vi "identity.vi"(8 "error in":errorcluster, 11 "Identity":T1 {"type" items=["Client", "Service"]}) -> (0 "error out":errorcluster, 3 "JSON Tree out (JSON Object)":variant)   [LabVIEW 2010]
uses:
  i3-json-1.0.0-10/JSON Generation/Create Value Files/Create Value - Object.vi
  i3-json-1.0.0-10/JSON Generation/Add Object Parameter Files/Add Object Parameter - String.vi
  i3-json-1.0.0-10/JSON Generation/Add Object Parameter Files/Add Object Parameter - Object.vi
  i3-json-1.0.0-10/i3-json.lvlib
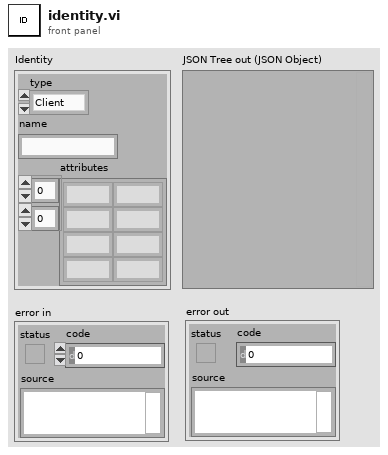
[diagram p1: front panel]
types:
  T1 = cluster{"type":u16, "name":string, "attributes":string[][]}
  T2 = enum32{"invalid CPU target", "Motorola 68K", "PowerPC", "Intel x86", "SPARC", "PA-RISC", "MIPS", "Alpha", "ARM", "AMD/Intel x64"}
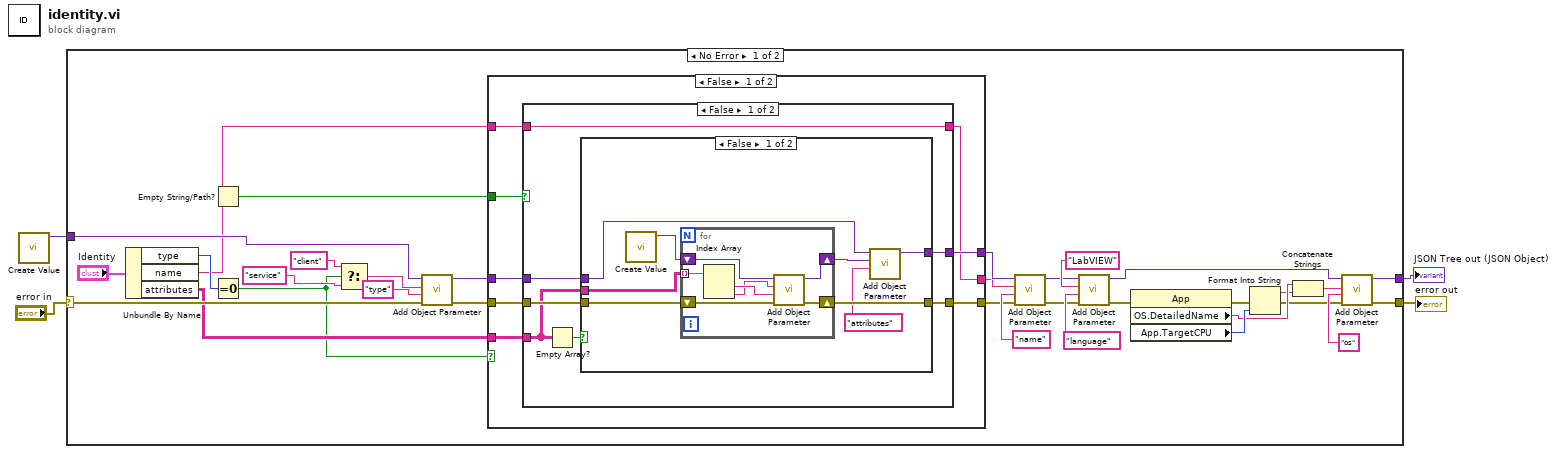
[diagram p0: block diagram]
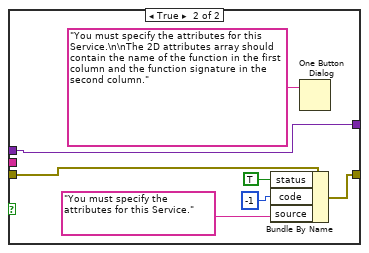
[diagram p2: hidden frame]
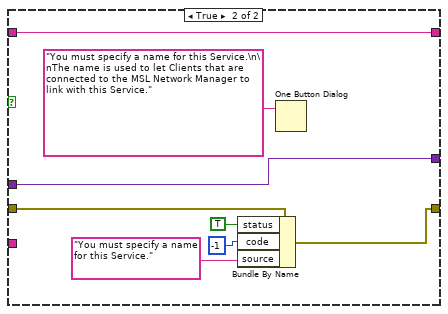
[diagram p3: hidden frame]
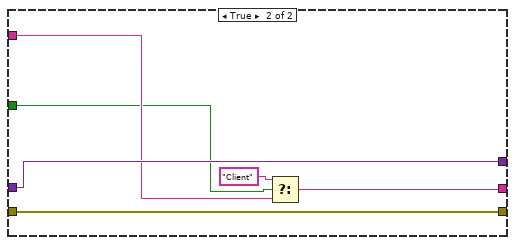
[diagram p4: hidden frame]
diagram:
  n1 = call-poly "Create Value.vi"() -> ("JSON Tree"=w3:variant)  [unwired: 10 in, 1 out]
  n2 = case shown="No Error" "error in" {
    selector: "error in" -> [w28 w90]
    tunnel: [w29 w89] -> w4
    tunnel: [w11 w90] -> w1
    tunnel: w3 -> [w27 w89]
    frame No Error {
      n3 = Unbundle By Name("Identity") -> ("type"=w26:u16, "name"=w8:string, "attributes"=w20:string[][])
      n4 = Empty String/Path?(string/path=w8) -> (empty?=w6:bool)
      n5 = Equal To 0?(x=w26) -> (x = 0?=w9:bool)
      n6 = Select(t="client" ("language"), s=w9, f="service") -> (s? t:f=w22:string)
      n7 = call-poly "Add Object Parameter.vi"("error in (no error)"=w28, "Name"="type", "String"=w22, "JSON Tree in (JSON Object)"=w27) -> ("error out"=w21:errorcluster, "JSON Tree out (JSON Object)"=w19:variant)  [unwired: 6 in]
      n8 = case shown="False" w9 {
        tunnel: [w42 w88] -> w17
        tunnel: w21 -> [w45 w88]
        tunnel: w20 -> [w43 _]
        tunnel: w19 -> [w44 w87]
        tunnel: [w41 w87] -> w18
        tunnel: w8 -> [w38 w85]
        tunnel: [w39 w84] -> w7
        tunnel: w6 -> [w40 w83]
        frame False {
          n9 = case shown="False" w40 {
            tunnel: w45 -> [w52 w79]
            tunnel: w44 -> [w51 w78]
            tunnel: w43 -> [w50 _]
            tunnel: [w48 w77] -> w42
            tunnel: [w47 w78] -> w41
            tunnel: [w46 w76] -> w39
            tunnel: w38 -> [w46 w76]
            frame False {
              n10 = Empty Array?(array=w50) -> (empty?=w49:bool)
              n11 = case shown="False" w49 {
                tunnel: w52 -> [w60 w73]
                tunnel: w51 -> [w56 w69]
                tunnel: w50 -> [w59 _]
                tunnel: [w58 w70] -> w48
                tunnel: [w53 w69] -> w47
                frame False {
                  n12 = call-poly "Create Value.vi"() -> ("JSON Tree"=w57:variant)  [unwired: 10 in, 1 out]
                  n13 = for {
                    tunnel: w59 -> [w63] mode=indexing
                    shift-right: [w66] -> w54
                    shift-left: w57 -> [w67]
                    shift-right: [w64] -> w58
                    shift-left: w60 -> [w65]
                    n14 = Index Array(array=w63) -> (element #1=w62:string, element #2=w61:string)  [unwired: 2 in]
                    n15 = call-poly "Add Object Parameter.vi"("error in (no error)"=w65, "Name"=w62, "String"=w61, "JSON Tree in (JSON Object)"=w67) -> ("error out"=w64:errorcluster, "JSON Tree out (JSON Object)"=w66:variant)  [unwired: 6 in]
                  }
                  n16 = call-poly "Add Object Parameter.vi"("Name"="attributes" ("String"), "JSON Object"=w54, "JSON Tree in (JSON Object)"=w56) -> ("JSON Tree out (JSON Object)"=w53:variant)  [unwired: 7 in, 1 out]
                }
                frame True {
                  n17 = Bundle By Name(cluster=w73, "status"=TRUE, "code"=-1, "source"="You must specify the attributes for this Service." ("message")) -> (w70:errorcluster)
                  n18 = One Button Dialog(message="You must specify the attributes for this Service.\n\nThe 2D attributes array should contain the name of the function in the first column and the function signature in the second column.") -> ()  [unwired: 1 in, 1 out]
                }
              }
            }
            frame True {
              n19 = Bundle By Name(cluster=w79, "status"=TRUE, "code"=-1, "source"="You must specify a name for this Service." ("message")) -> (w77:errorcluster)
              n20 = One Button Dialog(message="You must specify a name for this Service.\n\nThe name is used to let Clients that are connected to the MSL Network Manager to link with this Service.") -> ()  [unwired: 1 in, 1 out]
            }
          }
        }
        frame True {
          n21 = Select(t="Client" ("language"), s=w83, f=w85) -> (s? t:f=w84:string)
        }
      }
      n22 = call-poly "Add Object Parameter.vi"("error in (no error)"=w17, "Name"="name", "String"=w7, "JSON Tree in (JSON Object)"=w18) -> ("error out"=w13:errorcluster, "JSON Tree out (JSON Object)"=w15:variant)  [unwired: 6 in]
      n23 = call-poly "Add Object Parameter.vi"("error in (no error)"=w13, "Name"="language", "String"="LabVIEW" ("language"), "JSON Tree in (JSON Object)"=w15) -> ("error out"=w12:errorcluster, "JSON Tree out (JSON Object)"=w33:variant)  [unwired: 6 in]
      n24 = property class="App"(error in=w12) -> (error out=w14:errorcluster, "OS.DetailedName"=w30:string, "App.TargetCPU"=w32:T2)  [unwired: 1 in, 1 out]
      n25 = Format Into String(error in=w14, w32) -> (resulting string=w5:string, error out=w10:errorcluster)  [unwired: 2 in]
      n26 = Concatenate Strings(w30, w5) -> (w31:string)
      n27 = call-poly "Add Object Parameter.vi"("error in (no error)"=w10, "Name"="os", "String"=w31, "JSON Tree in (JSON Object)"=w33) -> ("error out"=w11:errorcluster, "JSON Tree out (JSON Object)"=w29:variant)  [unwired: 6 in]
    }
    frame Error {
    }
  }
  "JSON Tree out (JSON Object)" <- w4
  "error out" <- w1
